vi "Poll.vi"(7 "path override":path, 8 "error in (no error)":errorcluster, 9 "timeout_":i32, 10 "nitems_":i32, 11 "items_":T1) -> (0 "error out":errorcluster, 2 "function return":i32, 3 "items_ out":T1)   [LabVIEW 2025, in "LibZMQ.lvlib"]
doc: "ZMQ_EXPORT int zmq_poll (zmq_pollitem_t *items_, int nitems_, long timeout_);"
uses:
  LibZMQ.lvlib
  errno.vi
  strerror.vi
  <vilib>/Utility/error.llb/Error Cluster From Error Code.vi
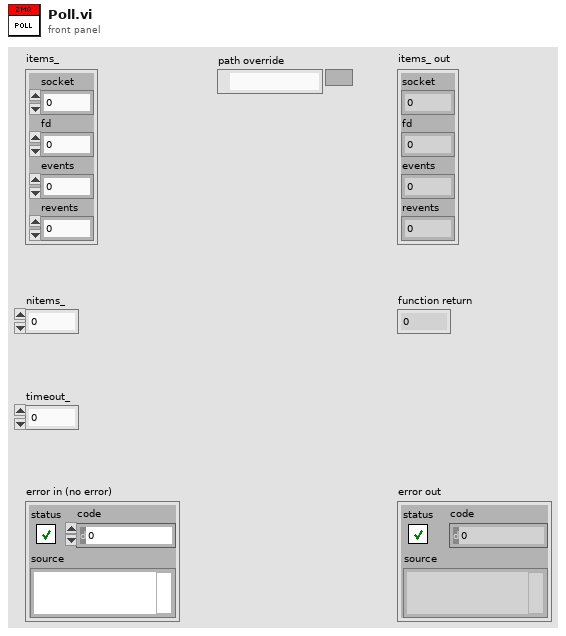
[diagram p1: front panel]
types:
  T1 = cluster{"socket":u32, "fd":i32, "events":i16, "revents":i16}
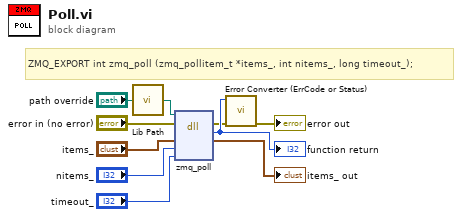
[diagram p0: block diagram]
diagram:
  # "ZMQ_EXPORT int zmq_poll (zmq_pollitem_t *items_, int nitems_, long timeout_);"
  n1 = call "Lib Path.vi"("path override"="path override") -> ("lib path"=w2:path)
  n2 = dll-call lib="libzmq-v143-mt-4_3_6.*" fn="zmq_poll"(path in=w2, error in="error in (no error)", "items_"="items_", "nitems_"="nitems_", "timeout_"="timeout_") -> (error out=w4:errorcluster, "return type"=w10:i32, "items_"=→"items_ out":T1)  [unwired: 3 in, 1 out]
  "function return" <- w10
  n3 = call "Error Converter (ErrCode or Status).vi"("error in (no error)"=w4, "error code"=w10) -> ("error out"=→"error out":errorcluster)  [unwired: 9 in]
